vi "PCO_GetSizes.vi"(8 "error in (no error)":errorcluster {"code" format="%x"}, 11 "ph":u64) -> (0 "error out":errorcluster {"code" format="%x"}, 1 "wXResAct":u16, 2 "ErrorMessage":i32 format="%x", 3 "ph out":u64, 4 "wXResMax":u16, 5 "wYResAct":u16, 7 "wYResMax":u16)   [LabVIEW 2019, in "SDK.lvlib" / "ImageSensor.lvlib"]
doc: "<b>Description:</b>\nThis function does return the current armed image size of the camera. If the user recently changed the size influencing values without issuing a PCO_ArmCamera, the PCO_GetSizes function will return the sizes from the last recording. If no recording occurred, it will return the last ROI settings. In case Soft ROI is enabled, PCO_GetSizes returns the sizes of the current Soft ROI. The values wXResAct and wYResAct return the current size, which should be used to allocate the buffers for image transfer. The values wXResMax and wYResMax return the maximum possible resolution including doubleshutter mode if available.\n\nPCO recommends the following order of commands: PCO_SetBinning, PCO_SetROI, PCO_ArmCamera, PCO_GetSizes and PCO_AllocateBuffer.\n\n<b>Supported camera type:</b>\nAll cameras\n\n<b>Descriptor dependency:</b>\nNone"
uses:
  ImageSensor.lvlib
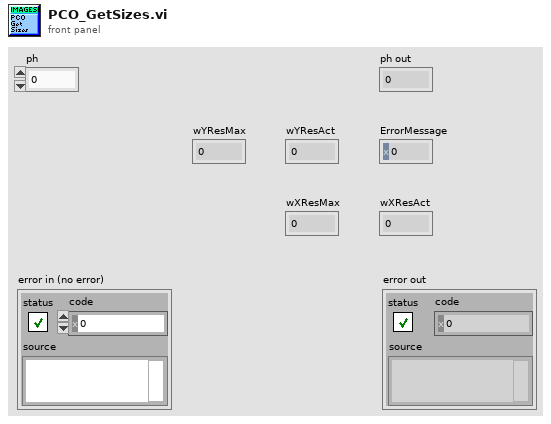
[diagram p1: front panel]
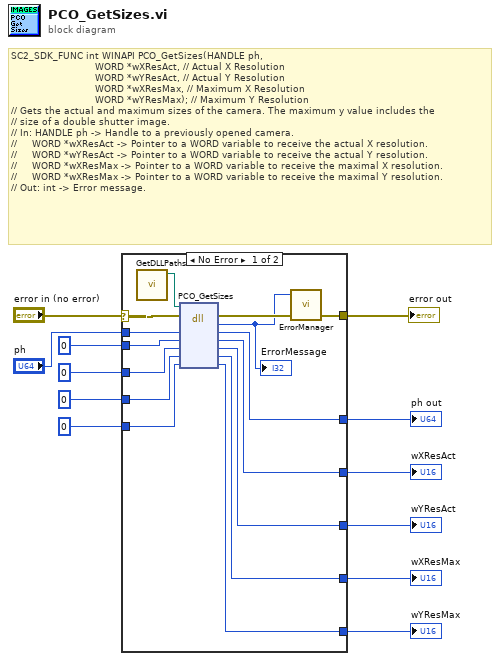
[diagram p0: block diagram]
diagram:
  # "SC2_SDK_FUNC int WINAPI PCO_GetSizes(HANDLE ph,\n                            WORD *wXResAct, // Actual X Resolution\n                            WORD *wYResAct, // Actual Y Resolution\n                            WORD *wXResMax, // Maximum X Resolution\n                            WORD *wYResMax); // Maximum Y Resolution\n// Gets the actual and maximum sizes of the camera. The maximum y value includes the\n// size of a double shutter image.\n// In: HANDLE ph -> Handle to a previously opened camera.\n//     WORD *wXResAct -> Pointer to a WORD variable to receive the actual X resolution.\n//     WORD *wYResAct -> Pointer to a WORD variable to receive the actual Y resolution.\n//     WORD *wXResMax -> Pointer to a WORD variable to receive the maximal X resolution.\n//     WORD *wXResMax -> Pointer to a WORD variable to receive the maximal Y resolution.\n// Out: int -> Error message."
  n1 = case shown="No Error" "error in (no error)" {
    selector: "error in (no error)" -> [w17 w28]
    tunnel: "ph" -> [w27 w33]
    tunnel: [w26 w33] -> w11
    tunnel: u16 0 ("wXResAct") -> [w25 w32]
    tunnel: [w24 w32] -> w9
    tunnel: u16 0 ("wYResAct") -> [w23 w31]
    tunnel: [w22 w31] -> w7
    tunnel: u16 0 ("wXResMax") -> [w21 w30]
    tunnel: [w20 w30] -> w5
    tunnel: u16 0 ("wYResMax") -> [w19 w29]
    tunnel: [w18 w29] -> w3
    tunnel: [w15 w28] -> w2
    frame No Error {
      n2 = call "GetDLLPaths.vi"() -> ("SC2_Cam_Path"=w13:path)  [unwired: 8 in, 3 out]
      n3 = dll-call lib="?" fn="PCO_GetSizes"(path in=w13, error in=w17, "ph"=w27, "wXResAct"=w25, "wYResAct"=w23, "wXResMax"=w21, "wYResMax"=w19) -> (error out=w16:errorcluster, "return type"=w14:i32, "ph"=w26:u64, "wXResAct"=w24:u16, "wYResAct"=w22:u16, "wXResMax"=w20:u16, "wYResMax"=w18:u16)  [unwired: 1 in, 1 out]
      "ErrorMessage" <- w14
      n4 = call "ErrorManager.vi"("error in (no error)"=w16, "error code"=w14) -> ("error out"=w15:errorcluster)  [unwired: 2 in, 1 out]
    }
    frame Error {
    }
  }
  "ph out" <- w11
  "wXResAct" <- w9
  "wYResAct" <- w7
  "wXResMax" <- w5
  "wYResMax" <- w3
  "error out" <- w2
